vi "Thermistor_Manual_Read.vi"(8 "error in":errorcluster, 9 "temp readings":T1, 11 "input cluster":T2={"Core"={"Current VI Reference"=refnum, "Close Panel on Exit?"=FALSE, "Exit"=FALSE, "Initialized?"=FALSE}, "Connections"={"cDAQ"={"Task"="", "Connected"=FALSE, "Active"=FALSE, "ID"=""}, "Camera"={"Session"="", "Connected"=FALSE, "Active"=FALSE, "Placeholder"=refnum}, "PSU"={"Port"="", "Connected"=FALSE, "Active"=FALSE}, "Arduino"={"Port"="", "Connected"=FALSE, "Active"=FALSE}}, "Data Acquisition"={"Setup"={"Label"="", "Operator"="", "Notes"="", "TempGrad"=1.0, "TargetTemp"=1.0, "Sample Volume"=1.0}, "Camera"={"Image"=refnum, "Save Image"=refnum, "Image Frequency"=20, "Rectangle"={"Left"=0, "Top"=0, "Right"=0, "Bottom"=0, "Rotation"=0.0}, "Calibration"={"Top Left"={"X"=0.0, "Y"=0.0}, "Top Right"={"X"=0.0, "Y"=0.0}, "Bottom Left"={"X"=0.0, "Y"=0.0}, "Bottom Right"={"X"=0.0, "Y"=0.0}, "Fixpoint"={"X"=0.0, "Y"=0.0}, "Scan Area"=0.0, "Fixpoint Area"=0.0, "Well Pixels"=[], "Valid"=FALSE}, "FocusPos"=0, "Display Mapping"=10, "Camera Mode"=10}, "Thermistor"={"Sample Size"=1, "Calibration"={"B0.100"=[], "R25"=[], "c"=[], "State"=[], "V_S"=5.0, "R_S"=100.0}, "Timing Mode"=14713}, "Partition"={"Data"=[], "Cell Label"="", "Cell Color"=0, "Height"=10, "Width"=16, "Grid"=[]}, "Queue"={"Size"=1, "Queue"=refnum}, "Sample Rate"=1, "Active"=FALSE, "Ready"=FALSE, "Graph Mode"=0, "Gradient Buffer"=2}, "Control"={"Sample Rate"=1, "PID gains"={"proportional gain (Kc)"=1.0, "integral time (Ti, min)"=0.01, "derivative time (Td, min)"=0.0}}, "Manual Temp Control"={"TargetTemp"=1.0, "Mode"=0, "Active"=FALSE}} {"Manual Temp Control"."Mode" items=["Cool", "Heat"]; "Manual Temp Control"."TargetTemp" min=-40.0 max=40.0 step=0.5 format="%#_g °C"; "Control"."PID gains"."derivative time (Td, min)" format="%.3f"; "Control"."PID gains"."integral time (Ti, min)" format="%.3f"; "Control"."PID gains"."proportional gain (Kc)" format="%.3f"; "Control"."Sample Rate" min=1 max=20 step=1 format="%.0f Samples/sec"; "Data Acquisition"."Gradient Buffer" min=2 max=30 step=1; "Data Acquisition"."Graph Mode" items=["Thermistor Temperature", "Camera Temperature"]; "Data Acquisition"."Thermistor"."Timing Mode" items=["Automatic"=16097, "High Resolution"=10195, "High Speed"=14712, "Best 50 Hz Rejection"=14713, "Best 60 Hz Rejection"=14714, "Custom"=10137]; "Data Acquisition"."Thermistor"."Calibration"."R_S" min=0.1 max=1000.0 format="%#_g kOhm"; "Data Acquisition"."Thermistor"."Calibration"."V_S" min=5.0 max=48.0 format="%#_g V"; "Data Acquisition"."Thermistor"."Calibration"."R25" min=0.1 max=1000.0 format="%#_g kOhm"; "Data Acquisition"."Thermistor"."Calibration"."B0.100" min=100.0 max=10000.0 format="%#_g K"; "Data Acquisition"."Thermistor"."Sample Size" min=1 max=200; "Data Acquisition"."Sample Rate" min=20 max=240 format="%.0f samples/min"; "Data Acquisition"."Queue"."Size" min=1 max=200; "Data Acquisition"."Camera"."Camera Mode" items=["Temperature Linear", "Signal Linear"]; "Data Acquisition"."Camera"."Display Mapping" items=["Default"=10, "Most Significant Bits"=11, "Full Dynamic"=12, "Downshift"=13, "Given Range"=14, "90% Dynamic"=15, "Given Percent Range"=16]; "Data Acquisition"."Camera"."Calibration"."Fixpoint"."Y" format="%.2f"; "Data Acquisition"."Camera"."Calibration"."Fixpoint"."X" format="%.2f"; "Data Acquisition"."Camera"."Calibration"."Top Left"."Y" format="%.2f"; "Data Acquisition"."Camera"."Calibration"."Top Left"."X" format="%.2f"; "Data Acquisition"."Camera"."Calibration"."Top Right"."Y" format="%.2f"; "Data Acquisition"."Camera"."Calibration"."Top Right"."X" format="%.2f"; "Data Acquisition"."Camera"."Calibration"."Bottom Left"."Y" format="%.2f"; "Data Acquisition"."Camera"."Calibration"."Bottom Left"."X" format="%.2f"; "Data Acquisition"."Camera"."Calibration"."Bottom Right"."Y" format="%.2f"; "Data Acquisition"."Camera"."Calibration"."Bottom Right"."X" format="%.2f"; "Data Acquisition"."Camera"."Rectangle"."Rotation" min=-90.0 max=90.0 step=1.0 format="%.2f"; "Data Acquisition"."Camera"."Rectangle"."Left" scale=0.0..1024.0; "Data Acquisition"."Camera"."Rectangle"."Right" scale=0.0..1024.0; "Data Acquisition"."Camera"."Image Frequency" min=1 max=60 step=1; "Data Acquisition"."Setup"."Sample Volume" min=0.0 max=500.0 format="%#_g µL"; "Data Acquisition"."Setup"."TargetTemp" min=-40.0 max=40.0 step=0.5 format="%#_g °C"; "Data Acquisition"."Setup"."TempGrad" min=-100.0 max=100.0 step=0.1 format="%#_g °C/min"}) -> (0 "error out":errorcluster, 3 "state":string)   [LabVIEW 2024]
uses:
  DataCluster.ctl
  <vilib>/userDefined/High Color/IMAQdx.ctl
  <vilib>/vision/Image Controls.llb/IMAQ Image.ctl
  <extravilib>/ChannelInstances/Tag-c(a[.](dbl),a[.](dbl))/))Channel.ctl
  <vilib>/Platform/TimedLoop/XDataNode/timing_clust.ctl
  <vilib>/Platform/TimedLoop/XDataNode/nitl_modes.ctl
  <vilib>/Platform/TimedLoop/XDataNode/wakeup.ctl
  <extravilib>/ChannelInstances/Tag-bool/Write With Abort.vi
  <extravilib>/ChannelInstances/Tag-c(a[.](dbl),a[.](dbl))/Read With Abort.vi
  <extravilib>/ChannelInstances/Tag-bool/Read With Abort.vi
  <extravilib>/ChannelInstances/Tag-bool/Instantiate.vi
  <extravilib>/ChannelInstances/Tag-c(a[.](dbl),a[.](dbl))/EndpointRead.vi
  <extravilib>/ChannelInstances/Tag-bool/EndpointRead.vi
  <extravilib>/ChannelInstances/Tag-bool/Endpoint.vi
  <vilib>/platform/TimedLoop/XDataNode/XDataNode.xnode
  <extravilib>/ChannelInstances/Tag-bool.lvlib
  <vilib>/Platform/TimedLoop/XDataNode/XDNodeRunTimeDep.lvlib
  <extravilib>/ChannelInstances/Tag-c(a[.](dbl),a[.](dbl)).lvlib
panel:
  out "T3":dbl caption="Temperature Probe 3" format="%.2f °C"
  out "T2":dbl caption="Temperature Probe 2" format="%.2f °C"
  out "T1":dbl caption="Temperature Probe 1" format="%.2f °C"
  out "Period (ms)":i64
  in  "Temp/Raw":enum32{"Temp", "Raw"}(radio)
  out "TRef":dbl caption="Reference Probe" format="%.2f °C"
  out "Status":string
  # "Primary Sensors"
  # "Additional Sensors"
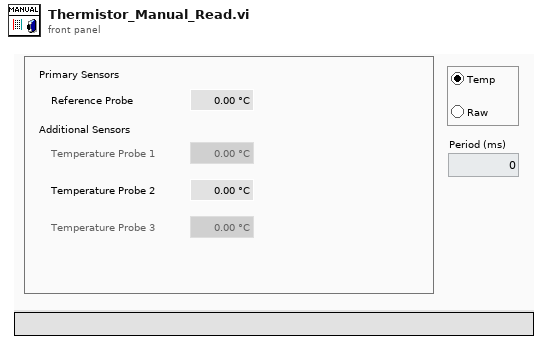
[diagram p1: front panel]
types:
  T1 = typedef "Tag-c(a[.](dbl),a[.](dbl)).lvlib/))Channel.ctl" = refnum<queue>
  T2 = typedef "DataCluster.ctl" = cluster{"Core":cluster{"Current VI Reference":refnum<vi>, "Close Panel on Exit?":bool, "Exit":bool, "Initialized?":bool}, "Connections":cluster{"cDAQ":cluster{"Task":refnum<k21>, "Connected":bool, "Active":bool, "ID":string}, "Camera":cluster{"Session":T3, "Connected":bool, "Active":bool, "Placeholder":T4}, "PSU":cluster{"Port":refnum<visa-resource-name>, "Connected":bool, "Active":bool}, "Arduino":cluster{"Port":refnum<visa-resource-name>, "Connected":bool, "Active":bool}}, "Data Acquisition":cluster{"Setup":cluster{"Label":string, "Operator":string, "Notes":string, "TempGrad":dbl, "TargetTemp":dbl, "Sample Volume":dbl}, "Camera":cluster{"Image":T4, "Save Image":T4, "Image Frequency":i32, "Rectangle":T5, "Calibration":cluster{"Top Left":T6, "Top Right":T6, "Bottom Left":T6, "Bottom Right":T6, "Fixpoint":T6, "Scan Area":dbl, "Fixpoint Area":dbl, "Well Pixels":cluster{"X":i32, "Y":i32}[][], "Valid":bool}, "FocusPos":u32, "Display Mapping":u32, "Camera Mode":u32}, "Thermistor":cluster{"Sample Size":i32, "Calibration":cluster{"B0.100":dbl[], "R25":dbl[], "c":dbl[][], "State":bool[], "V_S":dbl, "R_S":dbl}, "Timing Mode":i32}, "Partition":cluster{"Data":string[][], "Cell Label":string, "Cell Color":u32, "Height":i32, "Width":i32, "Grid":string[][]}, "Queue":cluster{"Size":i32, "Queue":refnum<queue>}, "Sample Rate":i32, "Active":bool, "Ready":bool, "Graph Mode":u16, "Gradient Buffer":i32}, "Control":cluster{"Sample Rate":i32, "PID gains":cluster{"proportional gain (Kc)":dbl, "integral time (Ti, min)":dbl, "derivative time (Td, min)":dbl}}, "Manual Temp Control":cluster{"TargetTemp":dbl, "Mode":u16, "Active":bool}}
  T3 = typedef "IMAQdx.ctl" = refnum<k21>
  T4 = typedef "IMAQ Image.ctl" = refnum<image>
  T5 = typedef "IMAQ Rectangle" = cluster{"Left":i32, "Top":i32, "Right":i32, "Bottom":i32, "Rotation":dbl}
  T6 = typedef "IMAQ Point" = cluster{"X":sgl, "Y":sgl}
  T7 = typedef "Tag-bool.lvlib/))Channel.ctl" = refnum<queue>
  T8 = enum8{"Enabled", "Disabled", "Disabled and Grayed Out"}
  T9 = typedef "XDNodeRunTimeDep.lvlib/timing_clust.ctl" = cluster{"Expected End [f-1]":u64, "Actual End [f-1]":u64, "Finished Late? [f-1]":bool, "Expected End [i-1]":u64, "Actual End [i-1]":u64, "Finished Late? [i-1]":bool, "Expected Start [i]":u64, "Actual Start [i]":u64, "Expected Start [f]":u64, "Actual Start [f]":u64, "Source Name":string, "Structure Name":string, "Period":i64, "Deadline":i64, "Offset":i64, "Start":i64, "Priority":i32, "Timeout":i32, "Mode":T10, "Wakeup Reason":T11, "Error":errorcluster, "Source Type":string, "Secondary Source Type":string, "Global End Time":u64, "Global Start Time":u64, "Frame Duration":u64, "Iteration Duration":u64, "Assigned CPU":i32, "I/O Scan Engine Mode":u32}
  T10 = typedef "XDNodeRunTimeDep.lvlib/nitl_modes.ctl" = enum32{"No Change", "Process missed periods, maintain original phase", "Discard missed periods, maintain original phase", "Process missed periods, ignore original phase", "Discard missed periods, ignore original phase"}
  T11 = typedef "XDNodeRunTimeDep.lvlib/wakeup.ctl" = enum32{"Normal", "Aborted", "Asynchronous wakeup", "Timing source error", "Timed loop error", "Timeout"}
  T12 = cluster{"Temperature Readings Duplicate":dbl[], "Voltage Readings Duplicate":dbl[]}
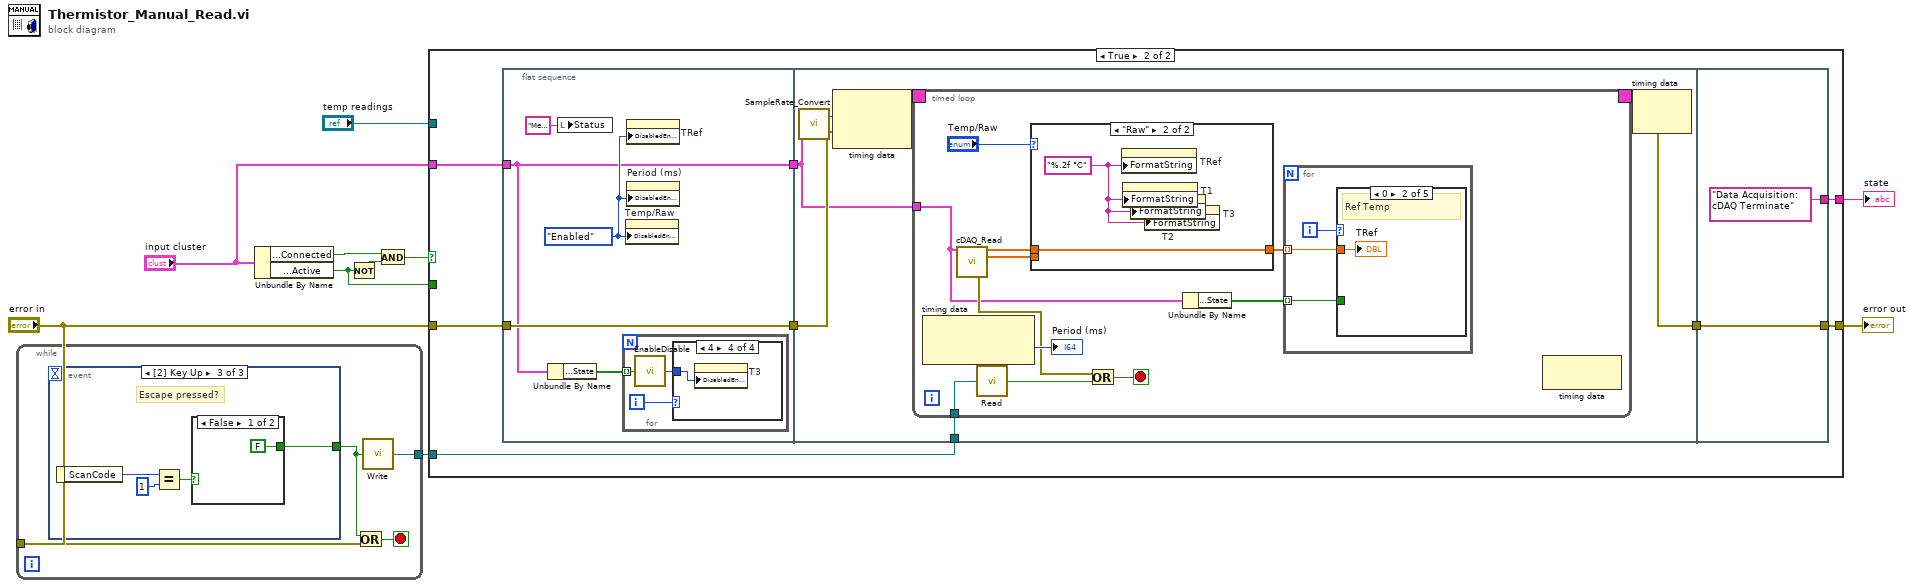
[diagram p0: block diagram]
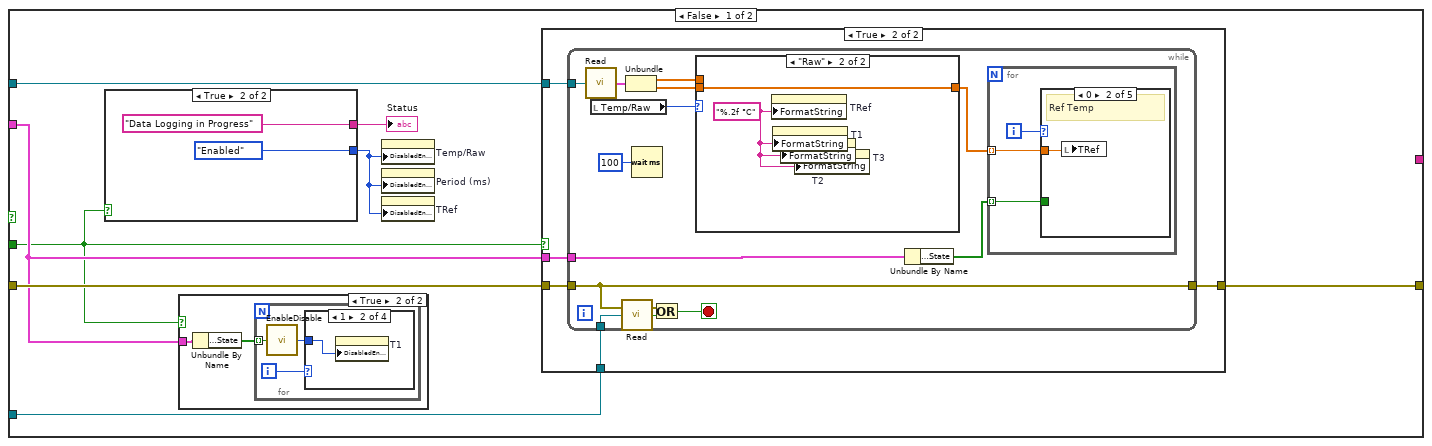
[diagram p2: hidden frame]
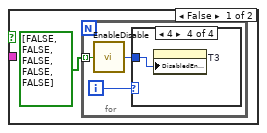
[diagram p3: hidden frame]
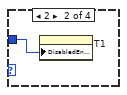
[diagram p5: hidden frame]
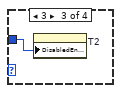
[diagram p6: hidden frame]
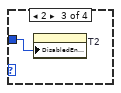
[diagram p8: hidden frame]
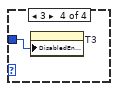
[diagram p9: hidden frame]
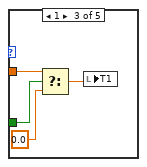
[diagram p12: hidden frame]
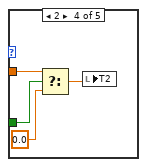
[diagram p13: hidden frame]
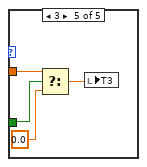
[diagram p14: hidden frame]
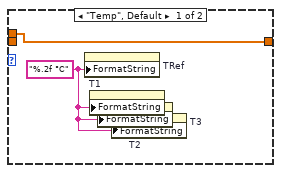
[diagram p15: hidden frame]
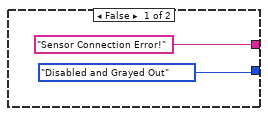
[diagram p16: hidden frame]
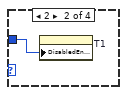
[diagram p18: hidden frame]
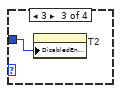
[diagram p19: hidden frame]
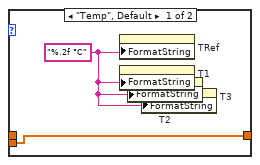
[diagram p20: hidden frame]
diagram:
  n1 = while {
    tunnel: "error in" -> [w12]
    tunnel: [w11] -> w7
    stop <- w13 stop-if-true
    n2 = event shown="[2] Key Up" {
      selector: _ -> [_ _ _]
      dyn-events: _ -> [_ _ _]
      timeout: _ -> [_ _ _]
      tunnel: [_ TRUE w19] -> w14
      event Timeout {
        n3 = event-data() -> ()  [unwired: 1 in, 1 out]
      }
      event Panel Close? {
        n4 = event-data() -> ()  [unwired: 1 in, 1 out]
        n5 = event-data() -> ()  [unwired: 2 in, 1 out]
      }
      event Key Up {
        # "Escape pressed?"
        n6 = event-data() -> ("ScanCode"=w18:i16)  [unwired: 1 in]
        n7 = Equal?(x=w18, y=i16 1) -> (x = y?=w16:bool)
        n8 = case shown="False" w16 {
          tunnel: [FALSE TRUE] -> w19
          frame False {
          }
          frame True {
          }
        }
      }
    }
    n9 = Or(x=w14, y=w12) -> (x .or. y?=w13:bool)
    n10 = call <extravilib>:"Write.vi"("element"=w14) -> ("channel"=w11:T7)  [unwired: 1 out]
  }
  n11 = Unbundle By Name("input cluster") -> ("Connections.cDAQ.Connected"=w10:bool, "Data Acquisition.Active"=w3:bool)
  n12 = Not(x=w3) -> (.not. x?=w4:bool)
  n13 = And(x=w10, y=w4) -> (x .and. y?=w5:bool)
  n14 = case shown="True" w5 {
    tunnel: "error in" -> [w27 w95]
    tunnel: [w24 w93] -> w9
    tunnel: w7 -> [w26 w91]
    tunnel: "input cluster" -> [w23 w89]
    tunnel: w3 -> [w22 _]
    tunnel: "temp readings" -> [w25 _]
    tunnel: [_ w88] -> w1
    frame False {
      n15 = case shown="True" w22 {
        tunnel: ["Sensor Connection Error!" ("String") "Data Logging in Progress" ("String")] -> w29
        tunnel: [T8."Disabled and Grayed Out" ("Disabled") T8."Enabled" ("Disabled")] -> w28
        frame False {
        }
        frame True {
        }
      }
      "Status" <- w29
      n16 = case shown="True" w22 {
        tunnel: w23 -> [_ w38]
        frame False {
          n17 = for {
            tunnel: bool[] [FALSE, FALSE, FALSE, FALSE, FALSE] ("State") -> [w32] mode=indexing
            i -> [w33]
            n18 = call "EnableDisable.vi"("EN?"=w32) -> ("Mode"=w31:T8)
            n19 = case shown="4" w33 {
              tunnel: w31 -> [_ w34 w35 w36]
              frame 0, Default {
              }
              frame 2 {
                n20 = property on="T1" class="DigNum (strict)"("DisabledEnum"=w34) -> ()  [unwired: 2 in, 2 out]
              }
              frame 3 {
                n21 = property on="T2" class="DigNum (strict)"("DisabledEnum"=w35) -> ()  [unwired: 2 in, 2 out]
              }
              frame 4 {
                n22 = property on="T3" class="DigNum (strict)"("DisabledEnum"=w36) -> ()  [unwired: 2 in, 2 out]
              }
            }
          }
        }
        frame True {
          n23 = Unbundle By Name(w38) -> ("Data Acquisition.Thermistor.Calibration.State"=w37:bool[])
          n24 = for {
            tunnel: w37 -> [w40] mode=indexing
            i -> [w41]
            n25 = call "EnableDisable.vi"("EN?"=w40) -> ("Mode"=w39:T8)
            n26 = case shown="1" w41 {
              tunnel: w39 -> [_ w42 w43 w44]
              frame 0, Default {
              }
              frame 1 {
                n27 = property on="T1" class="DigNum (strict)"("DisabledEnum"=w42) -> ()  [unwired: 2 in, 2 out]
              }
              frame 2 {
                n28 = property on="T2" class="DigNum (strict)"("DisabledEnum"=w43) -> ()  [unwired: 2 in, 2 out]
              }
              frame 3 {
                n29 = property on="T3" class="DigNum (strict)"("DisabledEnum"=w44) -> ()  [unwired: 2 in, 2 out]
              }
            }
          }
        }
      }
      n30 = property on="Temp/Raw" class="RadioBtnsControl (strict)"("DisabledEnum"=w28) -> ()  [unwired: 2 in, 2 out]
      n31 = property on="Period (ms)" class="DigNum (strict)"("DisabledEnum"=w28) -> ()  [unwired: 2 in, 2 out]
      n32 = property on="TRef" class="DigNum (strict)"("DisabledEnum"=w28) -> ()  [unwired: 2 in, 2 out]
      n33 = case shown="True" w22 {
        tunnel: w27 -> [w45 w50]
        tunnel: w26 -> [_ w49]
        tunnel: w25 -> [_ w48]
        tunnel: [w45 w47] -> w24
        tunnel: w23 -> [_ w46]
        frame False {
        }
        frame True {
          n34 = while {
            tunnel: w50 -> [w57]
            tunnel: w49 -> [w63]
            tunnel: w48 -> [w60]
            tunnel: [w57] -> w47
            tunnel: w46 -> [w51]
            stop <- w61 stop-if-true
            n35 = call <extravilib>:"Read.vi"("channel"=w60) -> ("element"=w59:T12)  [unwired: 1 in, 1 out]
            n36 = local read "Temp/Raw"() -> (w58:enum32{"Temp", "Raw"})
            n37 = call <extravilib>:"Read.vi"("channel"=w63) -> ("element"=w62:bool)  [unwired: 1 in, 1 out]
            n38 = Unbundle(w59) -> ("Temperature Readings Duplicate"=w56:dbl[], "Voltage Readings Duplicate"=w54:dbl[])
            n39 = Wait (ms)(milliseconds to wait=u32 100) -> ()  [unwired: 1 out]
            n40 = Or(x=w57, y=w62) -> (x .or. y?=w61:bool)
            n41 = case shown="\"Raw\"" w58 {
              tunnel: [w81 w83] -> w53
              tunnel: w54 -> [_ w83]
              tunnel: w56 -> [w81 _]
              frame "Temp", Default {
                w80 = "%.2f °C"
                n42 = property on="TRef" class="DigNum (strict)"("FormatString"=w80) -> ()  [unwired: 2 in, 2 out]
                n43 = property on="T1" class="DigNum (strict)"("FormatString"=w80) -> ()  [unwired: 2 in, 2 out]
                n44 = property on="T2" class="DigNum (strict)"("FormatString"=w80) -> ()  [unwired: 2 in, 2 out]
                n45 = property on="T3" class="DigNum (strict)"("FormatString"=w80) -> ()  [unwired: 2 in, 2 out]
              }
              frame "Raw" {
                w82 = "%.2f °C"
                n46 = property on="TRef" class="DigNum (strict)"("FormatString"=w82) -> ()  [unwired: 2 in, 2 out]
                n47 = property on="T1" class="DigNum (strict)"("FormatString"=w82) -> ()  [unwired: 2 in, 2 out]
                n48 = property on="T2" class="DigNum (strict)"("FormatString"=w82) -> ()  [unwired: 2 in, 2 out]
                n49 = property on="T3" class="DigNum (strict)"("FormatString"=w82) -> ()  [unwired: 2 in, 2 out]
              }
            }
            n50 = Unbundle By Name(w51) -> ("Data Acquisition.Thermistor.Calibration.State"=w52:bool[])
            n51 = for {
              tunnel: w53 -> [w65] mode=indexing
              tunnel: w52 -> [w64] mode=indexing
              i -> [w66]
              n52 = case shown="0" w66 {
                tunnel: w65 -> [_ w67 w70 w74 w78]
                tunnel: w64 -> [_ _ w71 w73 w77]
                frame -1, Default {
                }
                frame 0 {
                  # "Ref Temp"
                  n53 = local write "TRef"(w67) -> ()
                }
                frame 1 {
                  n54 = Select(t=w70, s=w71, f=0.0) -> (s? t:f=w68:dbl)
                  n55 = local write "T1"(w68) -> ()
                }
                frame 2 {
                  n56 = Select(t=w74, s=w73, f=0.0) -> (s? t:f=w72:dbl)
                  n57 = local write "T2"(w72) -> ()
                }
                frame 3 {
                  n58 = Select(t=w78, s=w77, f=0.0) -> (s? t:f=w76:dbl)
                  n59 = local write "T3"(w76) -> ()
                }
              }
            }
          }
        }
      }
    }
    frame True {
      n60 = flat-sequence {
        tunnel: w95 -> [w98]
        tunnel: [w98] -> w94
        tunnel: [w97] -> w90
        tunnel: w89 -> [w97]
        tunnel: w94 -> [w109]
        tunnel: [w108] -> w92
        tunnel: w91 -> [w113]
        tunnel: w90 -> [w107]
        tunnel: [w154] -> w93
        tunnel: w92 -> [w154]
        tunnel: ["Data Acquisition: cDAQ Terminate"] -> w88
        frame #0 {
          w99 = T8."Enabled" ("Disabled")
          n61 = Unbundle By Name(w97) -> ("Data Acquisition.Thermistor.Calibration.State"=w96:bool[])
          n62 = local write "Status"("Measurement Active!" ("Status")) -> ()
          n63 = for {
            tunnel: w96 -> [w102] mode=indexing
            i -> [w103]
            n64 = call "EnableDisable.vi"("EN?"=w102) -> ("Mode"=w101:T8)
            n65 = case shown="4" w103 {
              tunnel: w101 -> [_ w104 w105 w106]
              frame 0, Default {
              }
              frame 2 {
                n66 = property on="T1" class="DigNum (strict)"("DisabledEnum"=w104) -> ()  [unwired: 2 in, 2 out]
              }
              frame 3 {
                n67 = property on="T2" class="DigNum (strict)"("DisabledEnum"=w105) -> ()  [unwired: 2 in, 2 out]
              }
              frame 4 {
                n68 = property on="T3" class="DigNum (strict)"("DisabledEnum"=w106) -> ()  [unwired: 2 in, 2 out]
              }
            }
          }
          n69 = property on="Temp/Raw" class="RadioBtnsControl (strict)"("DisabledEnum"=w99) -> ()  [unwired: 2 in, 2 out]
          n70 = property on="TRef" class="DigNum (strict)"("DisabledEnum"=w99) -> ()  [unwired: 2 in, 2 out]
          n71 = property on="Period (ms)" class="DigNum (strict)"("DisabledEnum"=w99) -> ()  [unwired: 2 in, 2 out]
        }
        frame #1 {
          n72 = call "SampleRate_Convert.vi"("DataCluster"=w107) -> ("Sample dt (ms)"=w110:i64)  [unwired: 1 out]
          n73 = node-c288(w110, w109) -> (w112:T9)
          n74 = timed-loop {
            tunnel: w113 -> [w123]
            timing: w112 -> [_]
            timing-out: [_] -> w111
            tunnel: w107 -> [w116]
            stop <- w124 stop-if-true
            n75 = node-c288() -> (→"Period (ms)":i64)  [unwired: 1 in, 1 out]
            n76 = call "cDAQ_Read.vi"("DataCluster"=w116) -> ("Raw Readings"=w114:dbl[], "Temp Readings"=w118:dbl[], "error out"=w117:errorcluster)  [unwired: 7 in, 5 out]
            n77 = call <extravilib>:"Read.vi"("channel"=w123) -> ("element"=w122:bool)  [unwired: 1 in, 1 out]
            n78 = case shown="\"Raw\"" "Temp/Raw" {
              tunnel: w118 -> [w129 _]
              tunnel: [w129 w131] -> w120
              tunnel: w114 -> [_ w131]
              frame "Temp", Default {
                w128 = "%.2f °C"
                n79 = property on="TRef" class="DigNum (strict)"("FormatString"=w128) -> ()  [unwired: 2 in, 2 out]
                n80 = property on="T1" class="DigNum (strict)"("FormatString"=w128) -> ()  [unwired: 2 in, 2 out]
                n81 = property on="T2" class="DigNum (strict)"("FormatString"=w128) -> ()  [unwired: 2 in, 2 out]
                n82 = property on="T3" class="DigNum (strict)"("FormatString"=w128) -> ()  [unwired: 2 in, 2 out]
              }
              frame "Raw" {
                w130 = "%.2f °C"
                n83 = property on="TRef" class="DigNum (strict)"("FormatString"=w130) -> ()  [unwired: 2 in, 2 out]
                n84 = property on="T1" class="DigNum (strict)"("FormatString"=w130) -> ()  [unwired: 2 in, 2 out]
                n85 = property on="T2" class="DigNum (strict)"("FormatString"=w130) -> ()  [unwired: 2 in, 2 out]
                n86 = property on="T3" class="DigNum (strict)"("FormatString"=w130) -> ()  [unwired: 2 in, 2 out]
              }
            }
            n87 = Or(x=w117, y=w122) -> (x .or. y?=w124:bool)
            n88 = Unbundle By Name(w116) -> ("Data Acquisition.Thermistor.Calibration.State"=w115:bool[])
            n89 = for {
              tunnel: w120 -> [w133] mode=indexing
              tunnel: w115 -> [w132] mode=indexing
              i -> [w134]
              n90 = case shown="0" w134 {
                tunnel: w133 -> [_ w135 w138 w142 w145]
                tunnel: w132 -> [_ _ w139 w141 w144]
                frame -1, Default {
                }
                frame 0 {
                  # "Ref Temp"
                  "TRef" <- w135
                }
                frame 1 {
                  n91 = Select(t=w138, s=w139, f=0.0) -> (s? t:f=→"T1":dbl)
                }
                frame 2 {
                  n92 = Select(t=w142, s=w141, f=0.0) -> (s? t:f=→"T2":dbl)
                }
                frame 3 {
                  n93 = Select(t=w145, s=w144, f=0.0) -> (s? t:f=→"T3":dbl)
                }
              }
            }
            n94 = node-c288() -> ()  [unwired: 1 in, 1 out]
          }
          n95 = node-c288(w111) -> (w108:errorcluster)
        }
        frame #2 {
        }
      }
    }
  }
  "error out" <- w9
  "state" <- w1
